vi "Validate Licenece (unidirectional).vi"(8 "error in (no error)":errorcluster, 11 "licence key":string) -> (0 "error out":errorcluster, 3 "licence valid?":bool)   [LabVIEW 2013]
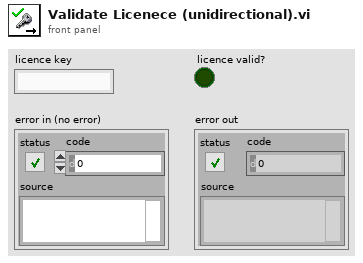
[diagram p1: front panel]
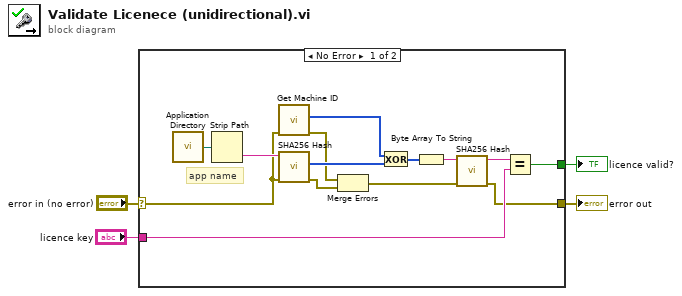
[diagram p0: block diagram]
diagram:
  n1 = case shown="No Error" "error in (no error)" {
    selector: "error in (no error)" -> [w5 w19]
    tunnel: [w12 _] -> w4
    tunnel: "licence key" -> [w7 _]
    tunnel: [w6 w19] -> w2
    frame No Error {
      # "app name"
      n2 = call <vilib>:"Application Directory.vi"() -> ("Application Directory"=w18:path)
      n3 = Strip Path(path=w18) -> (name=w11:string)  [unwired: 1 out]
      n4 = call "Get Machine ID.vi"("error in (no error)"=w5) -> ("error out"=w10:errorcluster, "machine ID bytes"=w15:u8[])  [unwired: 8 in, 1 out]
      n5 = call "SHA256 Hash.vi"("error in (no error)"=w5, "string to hash"=w11) -> ("error out"=w9:errorcluster, "hash bytes"=w16:u8[])  [unwired: 7 in, 1 out]
      n6 = Merge Errors(w10, w9) -> (w8:errorcluster)
      n7 = Exclusive Or(1:w16, 2:w15) -> (0:w14:u8[])
      n8 = Byte Array To String(unsigned byte array=w14) -> (string=w17:string)
      n9 = call "SHA256 Hash.vi"("error in (no error)"=w8, "string to hash"=w17) -> ("error out"=w6:errorcluster, "hex string hash"=w13:string)  [unwired: 7 in, 1 out]
      n10 = Equal?(x=w13, y=w7) -> (x = y?=w12:bool)
    }
    frame Error {
    }
  }
  "licence valid?" <- w4
  "error out" <- w2
